vi "Find Grippee.vi"(5 "Range":dbl, 7 "mm/pixel":dbl, 8 "picture":picture) -> (0 "picture":picture, 1 "mm/pixel":dbl, 2 "Range":dbl, 3 "result":cluster{"x":dbl, "y":dbl, "a":dbl})   [LabVIEW 2013]
uses:
  <vilib>/Analysis/baseanly.llb/Mean (DBL).vi
  <vilib>/Analysis/NI_AALPro.lvlib
  <vilib>/Analysis/NI_AALBase.lvlib
panel:
  in  "show?":bool=TRUE
  in  "Raw?":bool=TRUE
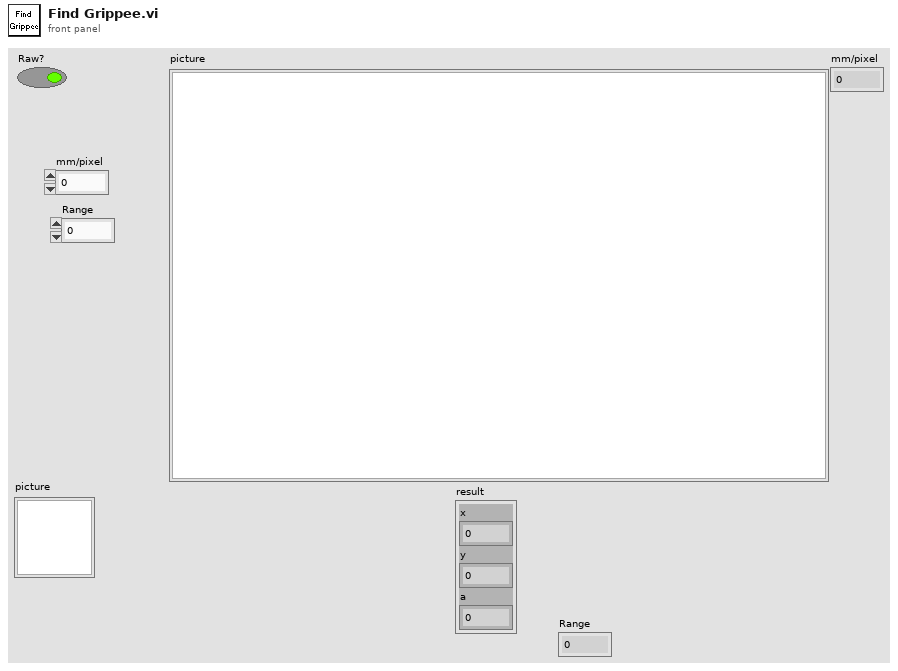
[diagram p1: front panel]
types:
  T1 = typedef "imagedata.ctl" = cluster{"image type":i32, "image depth":i32, "image":u8[], "mask":u8[], "colors":u32[], "Rectangle":cluster{"left":i16, "top":i16, "right":i16, "bottom":i16}}
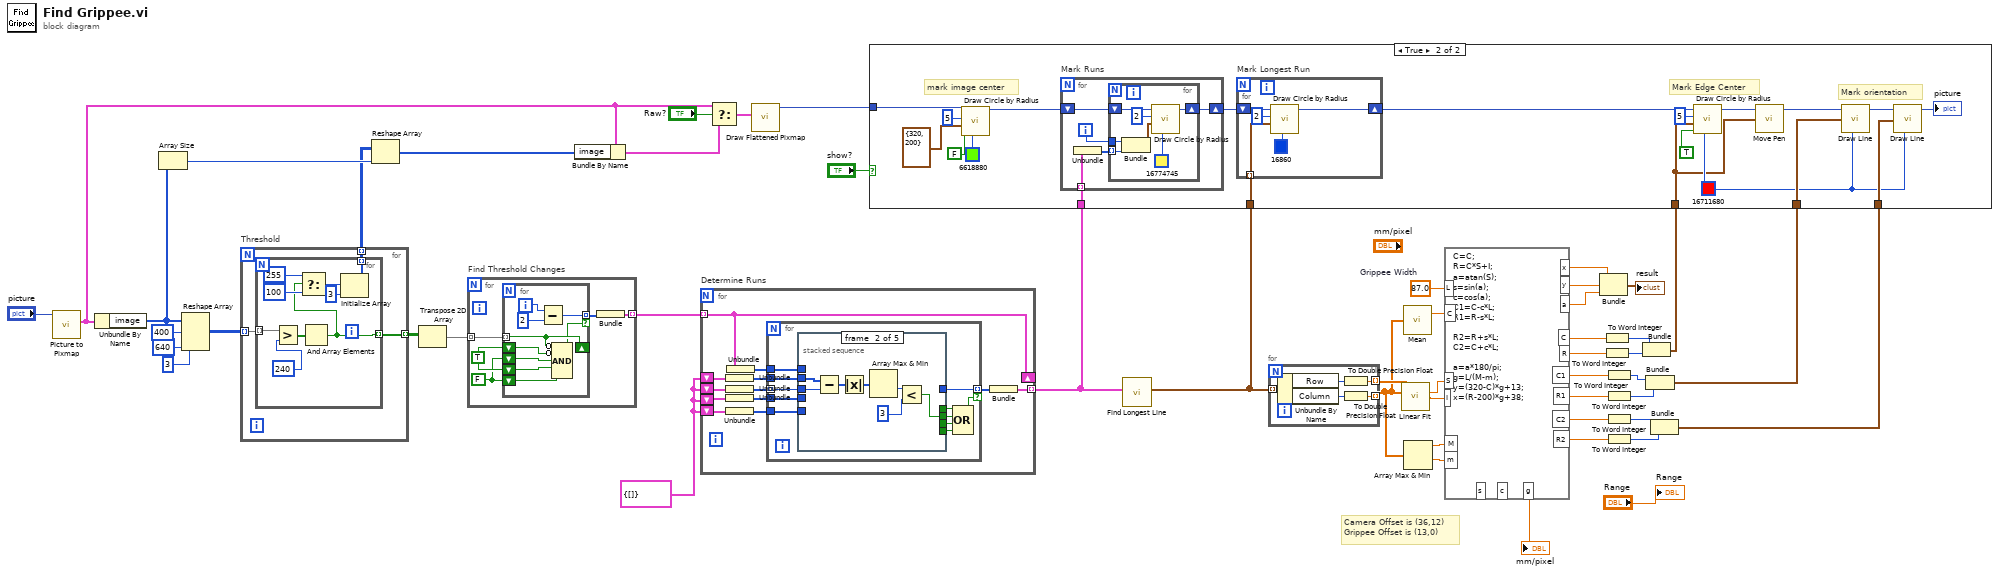
[diagram p0: block diagram]
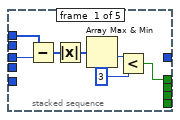
[diagram p3: hidden frame]
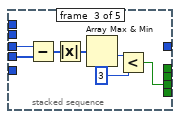
[diagram p4: hidden frame]
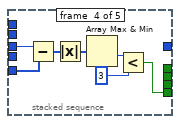
[diagram p5: hidden frame]
diagram:
  w31 = 87.0  # Grippee Width
  w33 = cluster{i32[]} {[]}
  # "Camera Offset is (36,12)\nGrippee Offset is (13,0)"
  n1 = call <vilib>:"Picture to Pixmap.vi"("picture"="picture") -> ("image data"=w40:T1)  [unwired: 9 in, 1 out]
  n2 = Unbundle By Name(w40) -> ("image"=w44:u8[])
  n3 = Array Size(array=w44) -> (size(s)=w45:i32)
  n4 = Reshape Array(w44, 400 ("dimension size"), 640 ("dimension size"), 3 ("dimension size")) -> (w38:u8[][][])
  n5 = for "Threshold" {
    tunnel: w38 -> [w53] mode=indexing
    tunnel: [w52] -> w36 mode=indexing
    tunnel: [w51] -> w37 mode=indexing
    n6 = for {
      tunnel: w53 -> [w54] mode=indexing
      tunnel: [w56] -> w52 mode=indexing
      tunnel: [w58] -> w51 mode=indexing
      n7 = Greater?(x=w54, y=u8 240) -> (0:w62:bool[])
      n8 = And Array Elements(Boolean array=w62) -> (logical AND=w56:bool)
      n9 = Select(t=u8 255, s=w56, f=u8 100) -> (s? t:f=w61:u8)
      n10 = Initialize Array(w61, 3 ("dimension size")) -> (w58:u8[])
    }
  }
  n11 = Reshape Array(w37, w45) -> (w46:u8[])
  n12 = Transpose 2D Array(2D array=w36) -> (transposed array=w35:bool[][])
  n13 = for "Find Threshold Changes" {
    tunnel: w35 -> [w67] mode=indexing
    tunnel: [w63] -> w34 mode=indexing
    w65 = FALSE
    w66 = TRUE
    n14 = for {
      tunnel: w67 -> [w74] mode=indexing
      shift-right: [w74] -> _
      shift-left: w66 -> [w73]
      shift-left: w65 -> [w72]
      shift-left: w66 -> [w71]
      shift-left: w65 -> [w70]
      tunnel: [w69] -> w64 mode=indexing if=w68
      i -> [w76]
      n15 = Subtract(x=w76, y=2) -> (x-y=w69:i32)
      n16 = Compound Arithmetic op=AND(invert w74, invert w73, w72, w71, w70) -> (w68:bool)
    }
    n17 = Bundle(w64) -> (w63:cluster{i32[]})  [unwired: 1 in]
  }
  n18 = Bundle By Name(cluster=w40, "image"=w46) -> (w43:T1)
  n19 = for "Determine Runs" {
    tunnel: w34 -> [w87] mode=indexing
    shift-right: [w87] -> _
    shift-left: w33 -> [w86]
    shift-left: w33 -> [w88]
    shift-left: w33 -> [w85]
    shift-left: w33 -> [w84]
    tunnel: [w83] -> w32 mode=indexing
    n20 = Unbundle(w86) -> (w78:i32[])
    n21 = Unbundle(w88) -> (w79:i32[])
    n22 = Unbundle(w85) -> (w80:i32[])
    n23 = Unbundle(w84) -> (w81:i32[])
    n24 = Unbundle(w87) -> (w77:i32[])
    n25 = for {
      tunnel: w79 -> [w98] mode=indexing
      tunnel: w77 -> [w99]
      tunnel: w78 -> [w97]
      tunnel: w80 -> [w93]
      tunnel: w81 -> [w91]
      tunnel: [w90] -> w82 mode=indexing if=w89
      n26 = stacked-sequence {
        tunnel: w99 -> [w106 _ _ _ _]
        tunnel: w98 -> [w105 w113 w115 w123 w128]
        tunnel: w97 -> [_ w108 _ _ _]
        tunnel: [_ w107 _ _ _] -> w96
        tunnel: [w100 _ _ _ _] -> w95
        tunnel: [_ _ w116 _ _] -> w94
        tunnel: w93 -> [_ _ w114 _ _]
        tunnel: [_ _ _ w122 _] -> w92
        tunnel: w91 -> [_ _ _ w121 _]
        tunnel: [_ _ _ _ w128] -> w90
        frame #0 {
          n27 = Subtract(x=w106, y=w105) -> (x-y=w104:i32[])
          n28 = Absolute Value(x=w104) -> (abs(x)=w103:i32[])
          n29 = Array Max & Min(array=w103) -> (min value=w102:i32)  [unwired: 3 out]
          n30 = Less?(x=w102, y=3) -> (x < y?=w100:bool)
        }
        frame #1 {
          n31 = Subtract(x=w108, y=w113) -> (x-y=w112:i32[])
          n32 = Absolute Value(x=w112) -> (abs(x)=w111:i32[])
          n33 = Array Max & Min(array=w111) -> (min value=w110:i32)  [unwired: 3 out]
          n34 = Less?(x=w110, y=3) -> (x < y?=w107:bool)
        }
        frame #2 {
          n35 = Subtract(x=w115, y=w114) -> (x-y=w120:i32[])
          n36 = Absolute Value(x=w120) -> (abs(x)=w119:i32[])
          n37 = Array Max & Min(array=w119) -> (min value=w118:i32)  [unwired: 3 out]
          n38 = Less?(x=w118, y=3) -> (x < y?=w116:bool)
        }
        frame #3 {
          n39 = Subtract(x=w123, y=w121) -> (x-y=w127:i32[])
          n40 = Absolute Value(x=w127) -> (abs(x)=w126:i32[])
          n41 = Array Max & Min(array=w126) -> (min value=w125:i32)  [unwired: 3 out]
          n42 = Less?(x=w125, y=3) -> (x < y?=w122:bool)
        }
        frame #4 {
        }
      }
      n43 = Compound Arithmetic op=OR(w95, w96, w94, w92) -> (w89:bool)
    }
    n44 = Bundle(w82) -> (w83:cluster{i32[]})  [unwired: 1 in]
  }
  n45 = Select(t=w40, s="Raw?", f=w43) -> (s? t:f=w42:T1)
  n46 = call <vilib>:"Draw Flattened Pixmap.vi"("image data"=w42) -> ("new picture"=w47:picture)  [unwired: 8 in]
  n47 = call "Find Longest Line.vi"("Array"=w32) -> ("Edge"=w9:cluster{"Column":i32, "Row":i32}[])  [unwired: 10 in]
  n48 = for {
    tunnel: w9 -> [w131] mode=indexing
    tunnel: [w130] -> w8 mode=indexing
    tunnel: [w129] -> w6 mode=indexing
    n49 = Unbundle By Name(w131) -> ("Row"=w132:i32, "Column"=w133:i32)
    n50 = To Double Precision Float(number=w132) -> (double precision float=w130:dbl)
    n51 = To Double Precision Float(number=w133) -> (double precision float=w129:dbl)
  }
  n52 = call <vilib>:"Linear Fit.vi"("Y"=w8, "X"=w6) -> ("slope"=w19:dbl, "intercept"=w18:dbl)  [unwired: 9 in, 3 out]
  n53 = call-poly <vilib>:"Mean.vi"("X"=w6) -> ("mean"=w20:dbl)  [unwired: 1 out]
  n54 = Array Max & Min(array=w6) -> (max value=w3:dbl, min value=w4:dbl)  [unwired: 2 out]
  n55 = formula code="C=C;\nR=C*S+I;\na=atan(S);\ns=sin(a);\nc=cos(a);\nC1=C-c*L;\nR1=R-s*L;\n\nR2=R+s*L;\nC2=C+c*L;\n\na=a*180/pi;\ng=L/(M-m);\ny=(320-C)*g+13;\nx=(R-200)*g+38;"("L"=w31, "C"=w20, "S"=w19, "I"=w18, "M"=w3, "m"=w4) -> ("C1"=w30:dbl, "R1"=w27:dbl, "C2"=w28:dbl, "R2"=w29:dbl, "a"=w10:dbl, "C"=w17:dbl, "R"=w16:dbl, "x"=w11:dbl, "y"=w12:dbl, "g"=→"mm/pixel":dbl)  [unwired: 2 out]
  n56 = Bundle("x"=w11, "y"=w12, "a"=w10) -> (→"result":cluster{"x":dbl, "y":dbl, "a":dbl})  [unwired: 1 in]
  n57 = To Word Integer(number=w17) -> (16bit integer=w15:i16)
  n58 = To Word Integer(number=w16) -> (16bit integer=w14:i16)
  n59 = To Word Integer(number=w30) -> (16bit integer=w26:i16)
  n60 = To Word Integer(number=w27) -> (16bit integer=w25:i16)
  n61 = To Word Integer(number=w28) -> (16bit integer=w23:i16)
  n62 = To Word Integer(number=w29) -> (16bit integer=w22:i16)
  n63 = Bundle(w15, w14) -> (w13:cluster{i16, i16})  [unwired: 1 in]
  n64 = Bundle(w26, w25) -> (w24:cluster{i16, i16})  [unwired: 1 in]
  n65 = Bundle(w23, w22) -> (w21:cluster{i16, i16})  [unwired: 1 in]
  n66 = case shown="True" "show?" {
    tunnel: w47 -> [_ w153]
    tunnel: w32 -> [_ w147]
    tunnel: w24 -> [_ w140]
    tunnel: w21 -> [_ w139]
    tunnel: w13 -> [_ w135]
    tunnel: w9 -> [_ w134]
    frame False {
    }
    frame True {
      w138 = u32 16711680
      # "Mark orientation"
      # "Mark Edge Center"
      # "mark image center"
      n67 = call <vilib>:"Draw Circle by Radius.vi"("color(black)"=u32 6618880, "fill?(F)"=FALSE, "pixel center"=cluster{"horizontal":i16, "vertical":i16} {"horizontal"=320, "vertical"=200}, "radius"=i16 5, "picture"=w153) -> ("new picture"=w146:picture)  [unwired: 6 in]
      n68 = for "Mark Runs" {
        shift-right: [w162] -> w145
        shift-left: w146 -> [w163]
        tunnel: w147 -> [w161] mode=indexing
        i -> [w159]
        n69 = Unbundle(w161) -> (w160:i32[])
        n70 = for {
          tunnel: w160 -> [w167] mode=indexing
          shift-right: [w169] -> w162
          shift-left: w163 -> [w170]
          tunnel: w159 -> [w165]
          n71 = Bundle(w165, w167) -> (w166:cluster{i32, i32})  [unwired: 1 in]
          n72 = call <vilib>:"Draw Circle by Radius.vi"("color(black)"=u32 16774745, "pixel center"=w166, "radius"=i16 2, "picture"=w170) -> ("new picture"=w169:picture)  [unwired: 7 in]
        }
      }
      n73 = for "Mark Longest Run" {
        shift-right: [w157] -> w144
        shift-left: w145 -> [w158]
        tunnel: w134 -> [w154] mode=indexing
        n74 = call <vilib>:"Draw Circle by Radius.vi"("color(black)"=u32 16860, "pixel center"=w154, "radius"=i16 2, "picture"=w158) -> ("new picture"=w157:picture)  [unwired: 7 in]
      }
      n75 = call <vilib>:"Draw Circle by Radius.vi"("color(black)"=w138, "fill?(F)"=TRUE, "pixel center"=w135, "radius"=i16 5, "picture"=w144) -> ("new picture"=w137:picture)  [unwired: 6 in]
      n76 = call <vilib>:"Move Pen.vi"("new position"=w135, "picture"=w137) -> ("new picture"=w136:picture)  [unwired: 3 in]
      n77 = call <vilib>:"Draw Line.vi"("picture"=w136, "end point"=w140, "color(black)"=w138) -> ("new picture"=w141:picture)  [unwired: 6 in]
      n78 = call <vilib>:"Draw Line.vi"("picture"=w141, "end point"=w139, "color(black)"=w138) -> ("new picture"=→"picture":picture)  [unwired: 6 in]
    }
  }
  "Range" <- "Range"
